vi "PWM_Cmd_v1.vi"(8 "error in (no error)":errorcluster, 9 "Duty Cycle":i32 min=0 max=100, 10 "Leg":i32 min=0 max=6, 11 "VISA Refnum in":refnum<visa-resource-name>) -> (0 "error out":errorcluster, 2 "Duty Cycle VISA Write":string, 3 "VISA Refnum out":refnum<visa-resource-name>)   [LabVIEW 2022 SP3]
panel:
  in  "Delay":dbl=0.1 format="%#_13g"
  out "read buffer":string
  out "Set Duty Cycle":string
  out ">":string
  out "Set PWM Leg":string
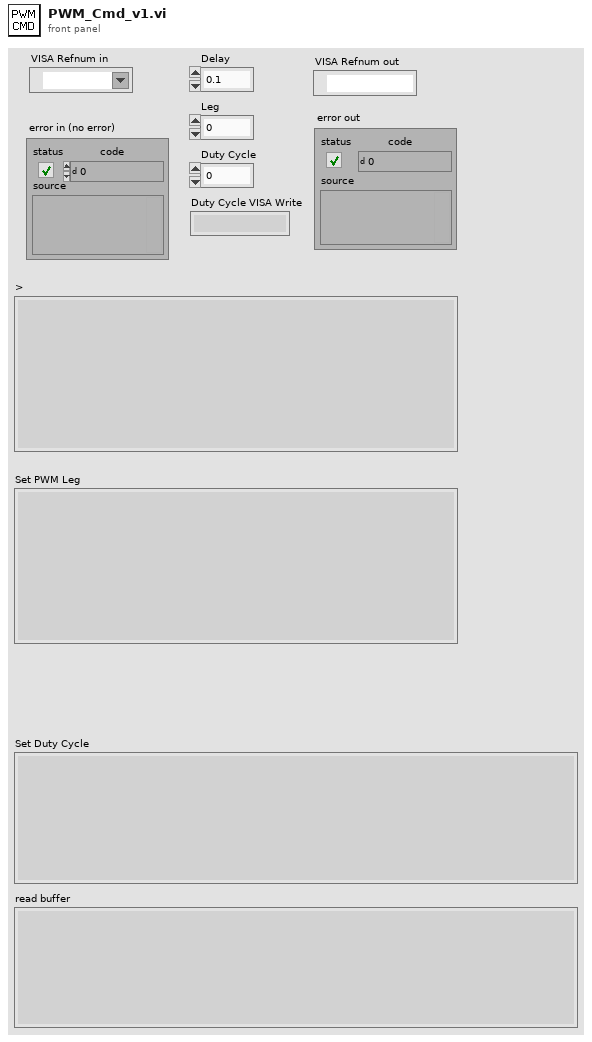
[diagram p1: front panel]
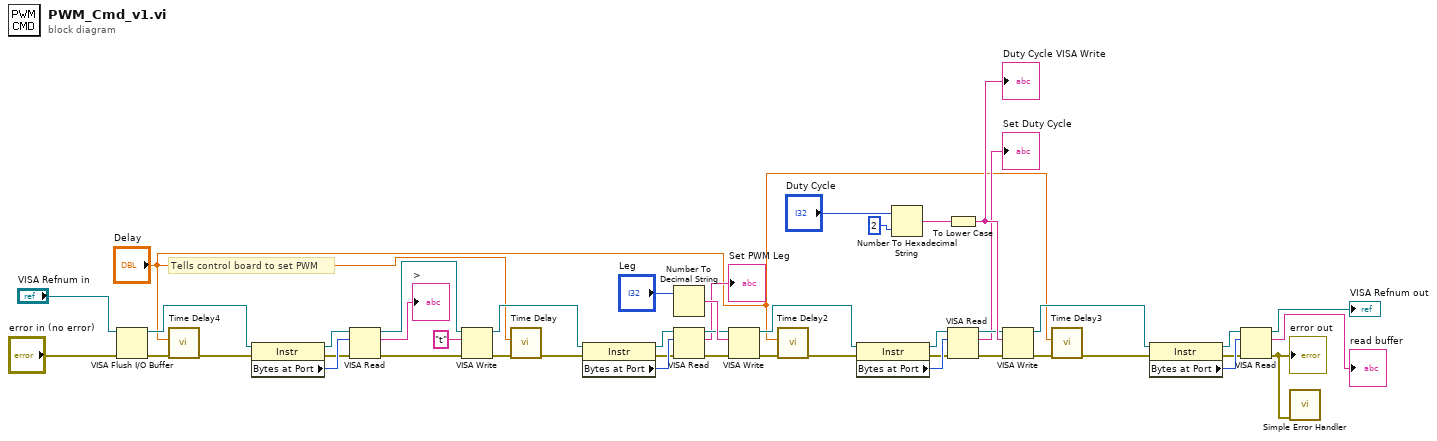
[diagram p0: block diagram]
diagram:
  # "Tells control board to set PWM"
  n1 = VISA Flush I/O Buffer(VISA resource name="VISA Refnum in", error in (no error)="error in (no error)") -> (VISA resource name out=w6:refnum<visa-resource-name>, error out=w3:errorcluster)  [unwired: 1 in]
  n2 = call "Time Delay4"("error in (no error)"=w3, "Delay Time (s)"="Delay") -> ("error out"=w2:errorcluster)  [unwired: 9 in]
  n3 = property class="Instr"(reference=w6, error in=w2) -> (reference out=w27:refnum<visa-resource-name>, error out=w7:errorcluster, "Bytes at Port"=w26:u32)
  n4 = VISA Read(VISA resource name=w27, byte count=w26, error in (no error)=w7) -> (VISA resource name out=w28:refnum<visa-resource-name>, read buffer=→">":string, error out=w29:errorcluster)  [unwired: 1 out]
  n5 = VISA Write(VISA resource name=w28, write buffer="t", error in (no error)=w29) -> (VISA resource name out=w41:refnum<visa-resource-name>, error out=w46:errorcluster)  [unwired: 1 out]
  n6 = call "Time Delay"("error in (no error)"=w46, "Delay Time (s)"="Delay") -> ("error out"=w24:errorcluster)  [unwired: 9 in]
  n7 = property class="Instr"(reference=w41, error in=w24) -> (reference out=w32:refnum<visa-resource-name>, error out=w23:errorcluster, "Bytes at Port"=w31:u32)
  n8 = Number To Decimal String(number="Leg") -> (decimal integer string=w35:string)  [unwired: 1 in]
  n9 = VISA Read(VISA resource name=w32, byte count=w31, error in (no error)=w23) -> (VISA resource name out=w34:refnum<visa-resource-name>, read buffer=→"Set PWM Leg":string, error out=w33:errorcluster)  [unwired: 1 out]
  n10 = VISA Write(VISA resource name=w34, write buffer=w35, error in (no error)=w33) -> (VISA resource name out=w40:refnum<visa-resource-name>, error out=w39:errorcluster)  [unwired: 1 out]
  n11 = call "Time Delay2"("error in (no error)"=w39, "Delay Time (s)"="Delay") -> ("error out"=w17:errorcluster)  [unwired: 9 in]
  n12 = property class="Instr"(reference=w40, error in=w17) -> (reference out=w21:refnum<visa-resource-name>, error out=w18:errorcluster, "Bytes at Port"=w20:u32)
  n13 = Number To Hexadecimal String(1:i16 2 ("width (-)"), 2:"Duty Cycle") -> (0:w43:string)
  n14 = To Lower Case(string=w43) -> (all lower case string=w42:string)
  "Duty Cycle VISA Write" <- w42
  n15 = VISA Read(VISA resource name=w21, byte count=w20, error in (no error)=w18) -> (VISA resource name out=w22:refnum<visa-resource-name>, read buffer=→"Set Duty Cycle":string, error out=w16:errorcluster)  [unwired: 1 out]
  n16 = VISA Write(VISA resource name=w22, write buffer=w42, error in (no error)=w16) -> (VISA resource name out=w44:refnum<visa-resource-name>, error out=w38:errorcluster)  [unwired: 1 out]
  n17 = call "Time Delay3"("error in (no error)"=w38, "Delay Time (s)"="Delay") -> ("error out"=w11:errorcluster)  [unwired: 9 in]
  n18 = property class="Instr"(reference=w44, error in=w11) -> (reference out=w14:refnum<visa-resource-name>, error out=w10:errorcluster, "Bytes at Port"=w13:u32)
  n19 = VISA Read(VISA resource name=w14, byte count=w13, error in (no error)=w10) -> (VISA resource name out=→"VISA Refnum out":refnum<visa-resource-name>, read buffer=→"read buffer":string, error out=w8:errorcluster)  [unwired: 1 out]
  "error out" <- w8
  n20 = call "Simple Error Handler.vi"("error in (no error)"=w8) -> ()  [unwired: 4 in, 5 out]
